vi "Test dZj(r,t) Graph.vi"() -> ()   [LabVIEW 2013, in "Zernike Polynome.lvlib"]
doc: "This VI is used to thest the radial behaviour of Zj(r,theta=const)."
uses:
  Zernike Polynome.lvlib
  <vilib>/Utility/NIReport.llb/NI_report.lvclass
  <vilib>/Analysis/coordinate.llb/3D Coordinate Conversion (Scalar).vi
  <vilib>/printing/ReportDocExtensions.llb/Append Front Panel Image to Report (path).vi
  <vilib>/Analysis/NI_AALPro.lvlib
  <vilib>/Platform/NI_3dgraph.lvlib
  <vilib>/Utility/NIReport.llb/NI_ReportGenerationCore.lvlib
panel:
  in  "X/Y":bool
  out "Time / ms":u32
  out "Time Graph":u32[](graph)
  out "dt / ms":u32
  in  "Show Graph?":bool
  in  "report file path":path
  in  "Print?":bool
  out "j":i32
  in  "Zj(r,theta) 3D Surface":refnum<k7>(container)
  in  "Nof Points":i32
  in  "j max":i32=100
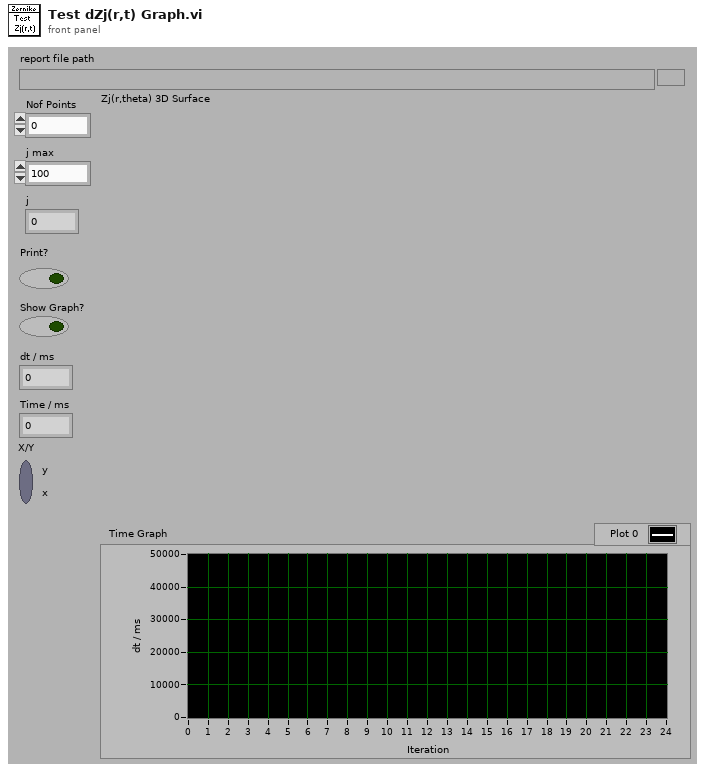
[diagram p1: front panel]
types:
  T1 = typedef "Zernike Polynome.lvlib/dZj(r,theta).ctl" = cluster{"dZj(r,theta)/dx":dbl, "dZj(r,theta)/dy":dbl}
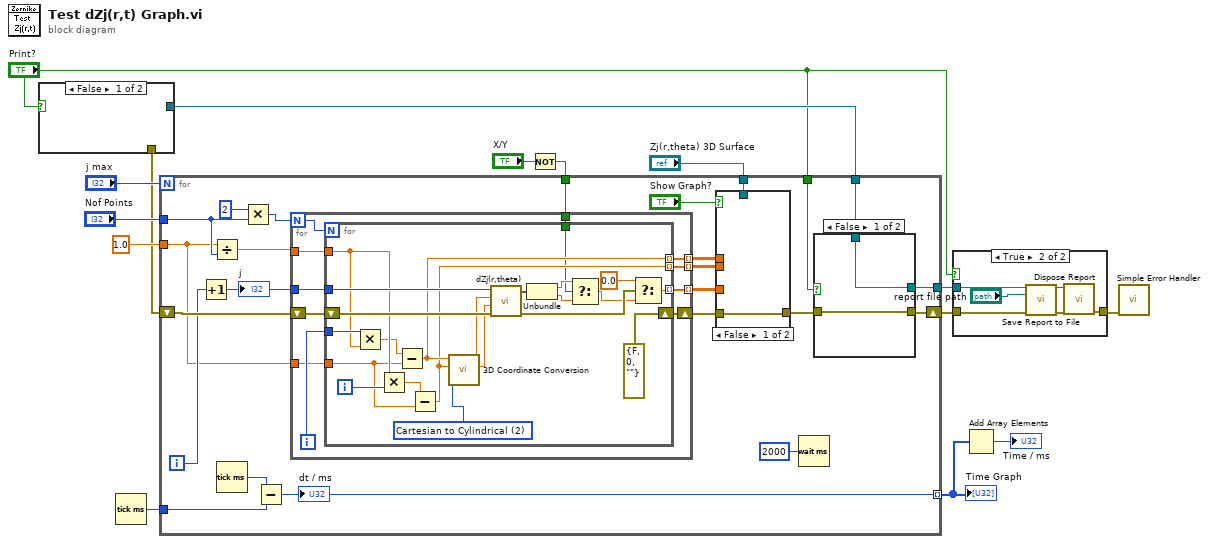
[diagram p0: block diagram]
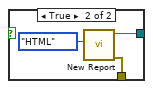
[diagram p3: hidden frame]
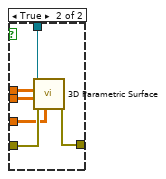
[diagram p4: hidden frame]
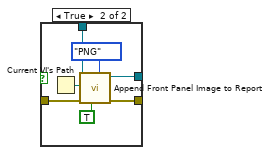
[diagram p5: hidden frame]
diagram:
  n1 = case shown="False" "Print?" {
    tunnel: [_ w17] -> w11
    tunnel: [_ w16] -> w10
    frame False {
    }
    frame True {
      n2 = call <vilib>:"New Report.vi"("report type"=enum16{"Standard Report", "HTML"}."HTML") -> ("report out"=w16:refnum<class "NI_report.lvclass">, "error out"=w17:errorcluster)  [unwired: 13 in]
    }
  }
  n3 = Tick Count (ms)() -> (millisecond timer value=w5:u32)
  n4 = Not(x="X/Y") -> (.not. x?=w2:bool)
  n5 = for {
    N: "j max" -> [_]
    tunnel: "Zj(r,theta) 3D Surface" -> [w42]
    tunnel: "Nof Points" -> [w35]
    shift-right: [w29] -> w8
    shift-left: w11 -> [w36]
    tunnel: 1.0 ("x") -> [w31]
    tunnel: w10 -> [w28]
    tunnel: [w27] -> w9
    tunnel: "Print?" -> [w26]
    tunnel: w5 -> [w23]
    tunnel: [w22] -> w4 mode=indexing
    tunnel: w2 -> [w20]
    i -> [w32]
    n6 = Increment(x=w32) -> (x+1=w21:i32)
    "j" <- w21
    n7 = Divide(x=w31, y=w35) -> (x/y=w39:dbl)
    n8 = Tick Count (ms)() -> (millisecond timer value=w24:u32)
    n9 = Multiply(x=2, y=w35) -> (x*y=w34:i32)
    n10 = Subtract(x=w24, y=w23) -> (x-y=w22:u32)
    "dt / ms" <- w22
    n11 = for {
      N: w34 -> [w66]
      shift-right: [w69] -> w41
      shift-left: w36 -> [w68]
      tunnel: w21 -> [w67]
      tunnel: [w65] -> w40 mode=indexing
      tunnel: w39 -> [w63]
      tunnel: [w62] -> w38 mode=indexing
      tunnel: [w61] -> w37 mode=indexing
      tunnel: w31 -> [w60]
      tunnel: w20 -> [w59]
      i -> [w64]
      n12 = for {
        N: w66 -> [_]
        shift-right: [errorcluster {"status"=FALSE, "code"=0, "source"=""} ("error out")] -> w69
        shift-left: w68 -> [w91]
        tunnel: w67 -> [w90]
        tunnel: [w77] -> w65 mode=indexing
        tunnel: w64 -> [w89]
        tunnel: w63 -> [w88]
        tunnel: [w82] -> w62 mode=indexing
        tunnel: [w80] -> w61 mode=indexing
        tunnel: w60 -> [w79]
        tunnel: w59 -> [w71]
        i -> [w87]
        w86 = u16 2 items=["Cartesian to Spherical", "Spherical to Cartesian", "Cartesian to Cylindrical", "Cylindrical to Cartesian", "Spherical to Cylindrical", "Cylindrical to Spherical"] ("conversion type")
        n13 = Multiply(x=w89, y=w88) -> (x*y=w83:dbl)
        n14 = Multiply(x=w88, y=w87) -> (x*y=w81:dbl)
        n15 = Subtract(x=w83, y=w79) -> (x-y=w82:dbl)
        n16 = Subtract(x=w81, y=w79) -> (x-y=w80:dbl)
        n17 = call-poly <vilib>:"3D Coordinate Conversion.vi"("conversion type"=w86, "axis 2"=w80, "axis 1"=w82) -> ("axis 2 out"=w84:dbl, "axis 1 out"=w85:dbl)  [unwired: 5 in, 2 out]
        n18 = call "dZj(r,theta).vi"("error in (no error)"=w91, "theta"=w84, "r"=w85, "j (1)"=w90) -> ("error out"=w78:errorcluster, "dZj(r,theta)"=w74:T1)  [unwired: 2 in]
        n19 = Unbundle(w74) -> ("dZj(r,theta)/dx"=w73:dbl, "dZj(r,theta)/dy"=w72:dbl)
        n20 = Select(t=w73, s=w71, f=w72) -> (s? t:f=w70:dbl)
        n21 = Select(t=0.0, s=w78, f=w70) -> (s? t:f=w77:dbl)
      }
    }
    n22 = case shown="False" "Show Graph?" {
      tunnel: w42 -> [_ w49]
      tunnel: w41 -> [w43 w48]
      tunnel: w40 -> [_ w47]
      tunnel: w38 -> [_ w46]
      tunnel: w37 -> [_ w45]
      tunnel: [w43 w44] -> w30
      frame False {
      }
      frame True {
        n23 = call <vilib>:"3D Parametric Surface.vi"("z matrix"=w47, "error in (no error)"=w48, "y matrix"=w45, "x matrix"=w46, "3D graph"=w49) -> ("error out"=w44:errorcluster)  [unwired: 5 in, 1 out]
      }
    }
    n24 = Wait (ms)(milliseconds to wait=u32 2000) -> ()  [unwired: 1 out]
    n25 = case shown="False" w26 {
      tunnel: w30 -> [w50 w58]
      tunnel: [w50 w57] -> w29
      tunnel: w28 -> [w51 w54]
      tunnel: [w51 w52] -> w27
      frame False {
      }
      frame True {
        n26 = Current VI's Path() -> (path=w55:path)
        n27 = call-poly <vilib>:"Append Front Panel Image to Report.vi"("report in"=w54, "image format (jpeg)"=enum32{"PNG", "JPEG", "GIF"}."PNG" ("Image Format (jpeg)"), "VI"=w55, "error in (no error)"=w58, "visible area only?"=TRUE) -> ("report out"=w52:refnum<class "NI_report.lvclass">, "error out"=w57:errorcluster)  [unwired: 6 in, 3 out]
      }
    }
  }
  "Time Graph" <- w4
  n28 = case shown="True" "Print?" {
    tunnel: w9 -> [_ w97]
    tunnel: w8 -> [w92 w96]
    tunnel: [w92 w98] -> w7
    frame False {
    }
    frame True {
      n29 = call-dynamic "Save Report to File.vi"("report in"=w97, "report file path"="report file path", "error in (no error)"=w96) -> ("report out"=w94:refnum<class "NI_report.lvclass">, "error out"=w95:errorcluster)  [unwired: 11 in]
      n30 = call-dynamic "Dispose Report.vi"("report in"=w94, "error in (no error)"=w95) -> ("error out"=w98:errorcluster)  [unwired: 13 in]
    }
  }
  n31 = Add Array Elements(numeric array=w4) -> (sum=→"Time / ms":u32)
  n32 = call <vilib>:"Simple Error Handler.vi"("error in (no error)"=w7) -> ()  [unwired: 4 in, 5 out]
